vi "Write GUID.vi"(8 "error in (no error)":errorcluster, 10 "GUID":string, 11 "Launch Functions Message in":refnum<class "Launch Functions Message.lvclass">) -> (0 "error out":errorcluster, 3 "Launch Functions Message out":refnum<class "Launch Functions Message.lvclass">)   [LabVIEW 2016, in "Controller Actor.lvlib" / "Launch Functions Message.lvclass"]
uses:
  <userlib>/Common Components/Controller/Messages/Launch Functions Message/Launch Functions Message.lvclass
  <userlib>/Common Components/Controller/Messages/Launch Functions Message/Launch Functions Message.lvclass/Launch Functions Message.ctl
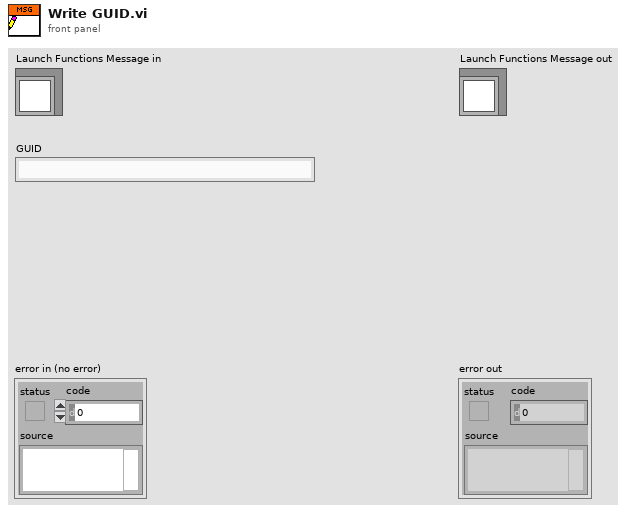
[diagram p1: front panel]
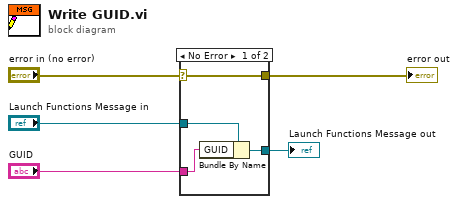
[diagram p0: block diagram]
diagram:
  n1 = case shown="No Error" "error in (no error)" {
    selector: "error in (no error)" -> [w9 w10]
    tunnel: [w9 w10] -> w4
    tunnel: [w7 w11] -> w2
    tunnel: "Launch Functions Message in" -> [w8 w11]
    tunnel: "GUID" -> [w6 _]
    frame No Error {
      n2 = Bundle By Name(cluster=w8, "GUID"=w6) -> (w7:refnum<class "Launch Functions Message.lvclass">)
    }
    frame Error {
    }
  }
  "error out" <- w4
  "Launch Functions Message out" <- w2
